vi "FtoC.vi"() -> ()   [LabVIEW 2009]
panel:
  out "CELCIUS(C)":dbl(slide) scale=0.0..100.0
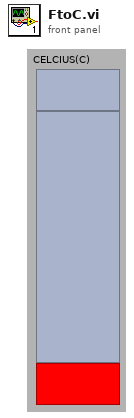
[diagram p1: front panel]
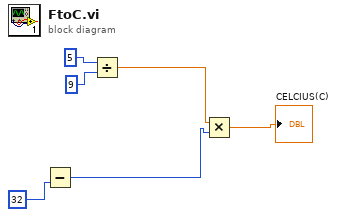
[diagram p0: block diagram]
diagram:
  n1 = Subtract(y=32) -> (x=w7:i32, x-y=w1:i32)
  n2 = Divide(x=5, y=9) -> (x/y=w6:dbl)
  n3 = Multiply(x=w6, y=w1) -> (x*y=→"CELCIUS(C)":dbl)
